vi "AbsPositionToPicture.vi"(10 "input position":cluster{"X":dbl, "Y":dbl, "Angle":dbl}) -> (2 "output point":cluster{"x":i16, "y":i16})   [LabVIEW 2009, in "Host.lvlib" / "Draw.lvlib"]
uses:
  Draw.lvlib
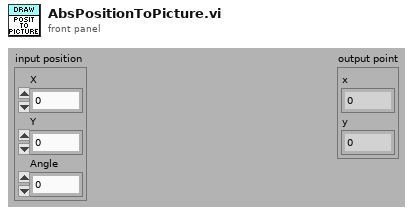
[diagram p1: front panel]
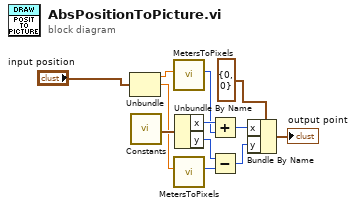
[diagram p0: block diagram]
diagram:
  n1 = Unbundle("input position") -> ("X"=w4:dbl, "Y"=w6:dbl)  [unwired: 1 out]
  n2 = call "Constants.vi"() -> ("PictureCenterPoint"=w7:cluster{"x":i16, "y":i16})  [unwired: 16 in, 3 out]
  n3 = call "MetersToPixels.vi"("meters"=w4) -> ("pixels"=w3:i32)  [unwired: 10 in]
  n4 = call "MetersToPixels.vi"("meters"=w6) -> ("pixels"=w5:i32)  [unwired: 10 in]
  n5 = Unbundle By Name(w7) -> ("x"=w11:i16, "y"=w9:i16)
  n6 = Add(x=w11, y=w3) -> (x+y=w10:i32)
  n7 = Subtract(x=w9, y=w5) -> (x-y=w8:i32)
  n8 = Bundle By Name(cluster=cluster{"x":i16, "y":i16} {"x"=0, "y"=0} ("end point"), "x"=w10, "y"=w8) -> (→"output point":cluster{"x":i16, "y":i16})
